vi "JSONBoolean.vi"() -> ()   [LabVIEW 2023]
uses:
  <vilib>/JDP Science/JSONtext/JSONtext.lvlib
  81b0af02-4781-4b57-905b-31a708286598.vi
  AcquisitionReady.ctl
  CCD.lvclass
panel:
  out "Data out":T1
  out "<JSON>":string caption="<JSON>Item"
  out "ready":bool
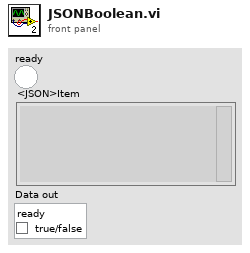
[diagram p1: front panel]
types:
  T1 = typedef "CCD.lvclass/AcquisitionReady.ctl" = cluster{"ready":bool}
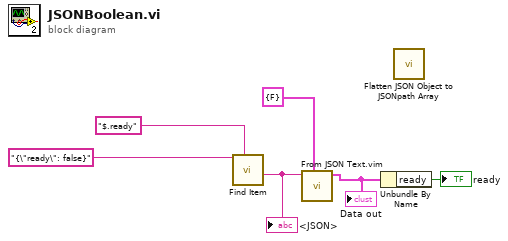
[diagram p0: block diagram]
diagram:
  n1 = call <vilib>:"Find Item.vi"("$Path or Item Name"="$.ready", "JSON"="{\"ready\": false}") -> ("<JSON>"=w4:string)  [unwired: 6 in, 3 out]
  "<JSON>" <- w4
  n2 = call "From JSON Text.vim"("Data Type and Default Value"=T1 {"ready"=FALSE} ("ccd acquisition ready?"), "JSON"=w4) -> ("Data out"=w3:T1)  [unwired: 8 in, 1 out]
  "Data out" <- w3
  n3 = Unbundle By Name(w3) -> ("ready"=→"ready":bool)
  n4 = call <vilib>:"Flatten JSON Object to JSONpath Array.vi"() -> ()  [unwired: 9 in, 3 out]
